vi "synchronization_prototype.vi"() -> ()   [LabVIEW 2015]
uses:
  <vilib>/userdefined/High Color/nirio_resource_hc.ctl
  FPGA_Controls/trigger_channel.ctl
  <vilib>/DAQmx/read.llb/DAQmx Read (Analog Wfm 1Chan NSamp).vi
  <vilib>/Utility/error.llb/Error Cluster From Error Code.vi
  <vilib>/rvi/errors/niLvFpgaAdjustHostInterfaceError.vi
  <vilib>/DAQmx/create/channels.llb/DAQmx Create Channel (AI-Voltage-Basic).vi
  <vilib>/DAQmx/configure/timing.llb/DAQmx Timing (Sample Clock).vi
  <vilib>/DAQmx/create/channels.llb/DAQmx Create Channel (CO-Pulse Generation-Time).vi
  <vilib>/DAQmx/configure/timing.llb/DAQmx Timing (Implicit).vi
  <vilib>/DAQmx/configure/trigger.llb/DAQmx Start Trigger (Digital Edge).vi
  <instrlib>/niSync/niSync.llb/niSync Initialize (IVI).vi
  <vilib>/DAQmx/miscellaneous.llb/DAQmx Fill In Error Info.vi
  <vilib>/FPGAPlugInAG/Dynamic/niLvFpga_Close_Dynamic.vi
  <vilib>/rvi/interface/nirviReadWriteControl/nirviReadWriteControl.xnode
  <vilib>/rvi/interface/nirviCloseFPGA/nirviCloseFPGA.xnode
  <resource>/objmgr/daqmx.rc
  <vilib>/rvi/interface/Simulation/niFpgaSimulationCallBeginRW.vi
  NiFpgaLv.dll
panel:
  in  "Pulse delay":dbl=1e-05 format="%#_13g"
  in  "Pulse counter destination terminal":string(combo)="PXI_Trig1"
  in  "DAQ pulse gen looking at:":tag
  in  "DAQ pulse gen counter":tag
  in  "DAQ Physical Channel":tag
  in  "samples DAQ":i32=1000
  in  "FPGA AI to plot":i32
  out "RIO":waveform(dbl)(graph)
  out "Interleaved Raw Data":u64[](array[numeric])
  out "Counts":i16[][](array[numeric])
  out "Voltage":dbl[][](array[numeric])
  in  "Trigger Channel FPGA looks at":T1
  in  "FPGA delay (x 50ns)":u64
  in  "num samples RIO":u64=1000
  in  "FPGA name":T2 caption="RIO Device"
  out "DAQ":waveform(dbl)(graph)
  in  "DAQ listens to":tag
  in  "DAQ Delay (s)":dbl
  in  "RIO Destination Terminal":string(combo)="PXI_Trig1"
  in  "DAQ destination terminal":string(combo)="PXI_Trig1"
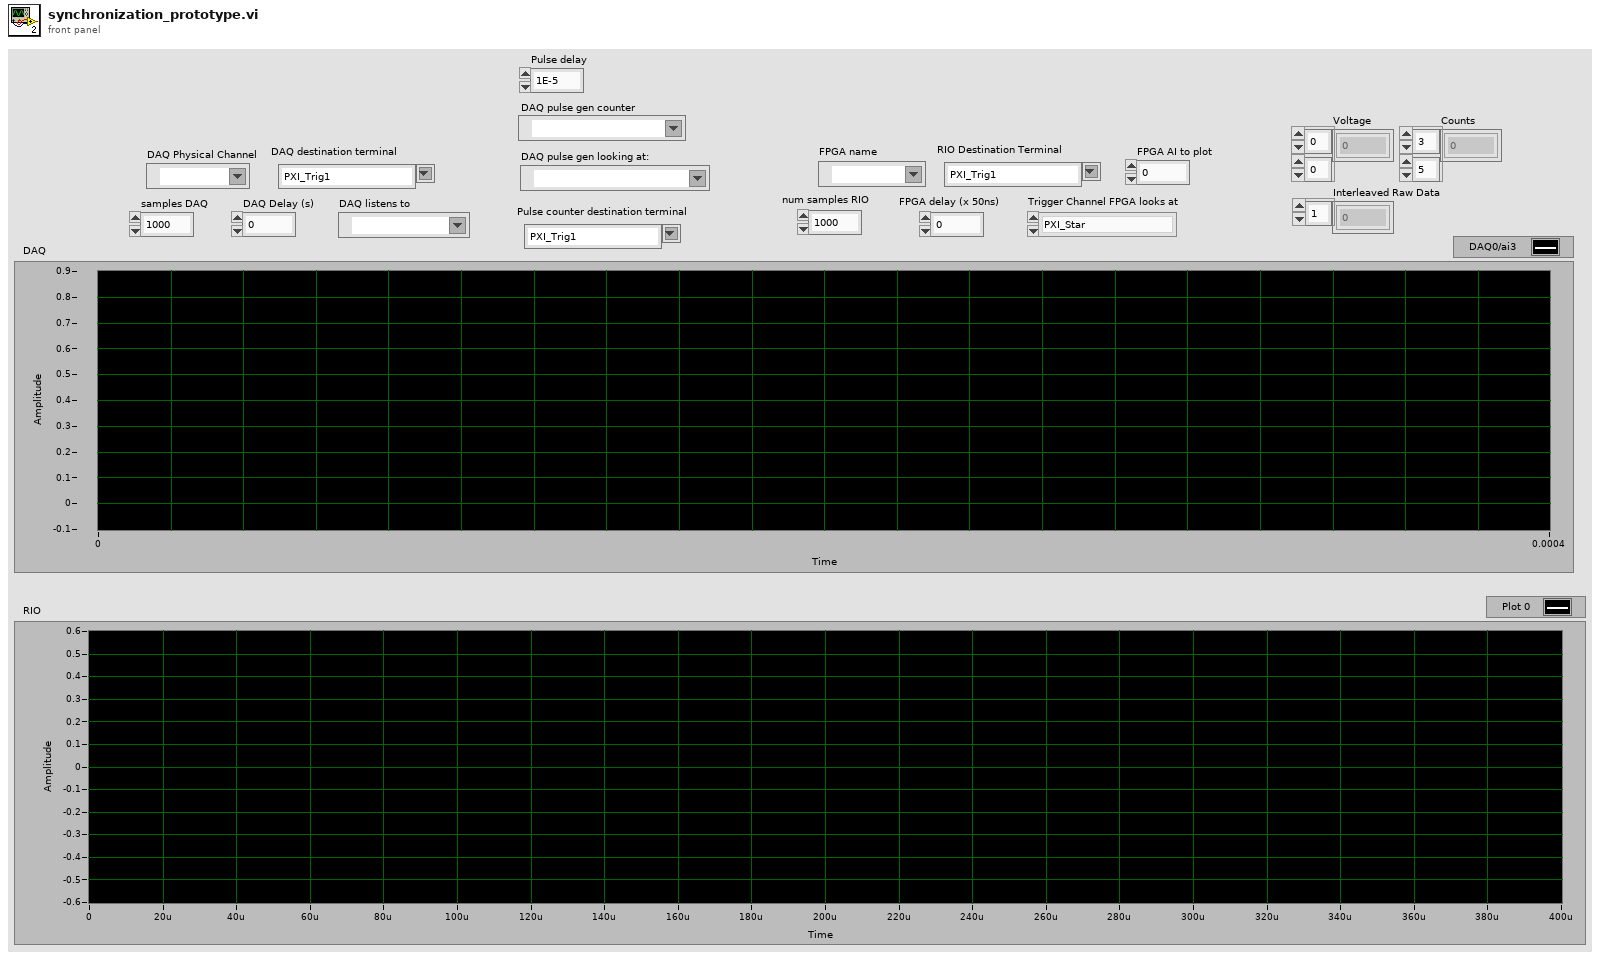
[diagram p1: front panel]
types:
  T1 = typedef "trigger_channel.ctl" = enum16{"PXI_Star", "PXI_Trig0", "PXI_Trig1", "PXI_Trig2", "PXIe_DStarB", "False", "True"}
  T2 = typedef "nirio_resource_hc.ctl" = tag
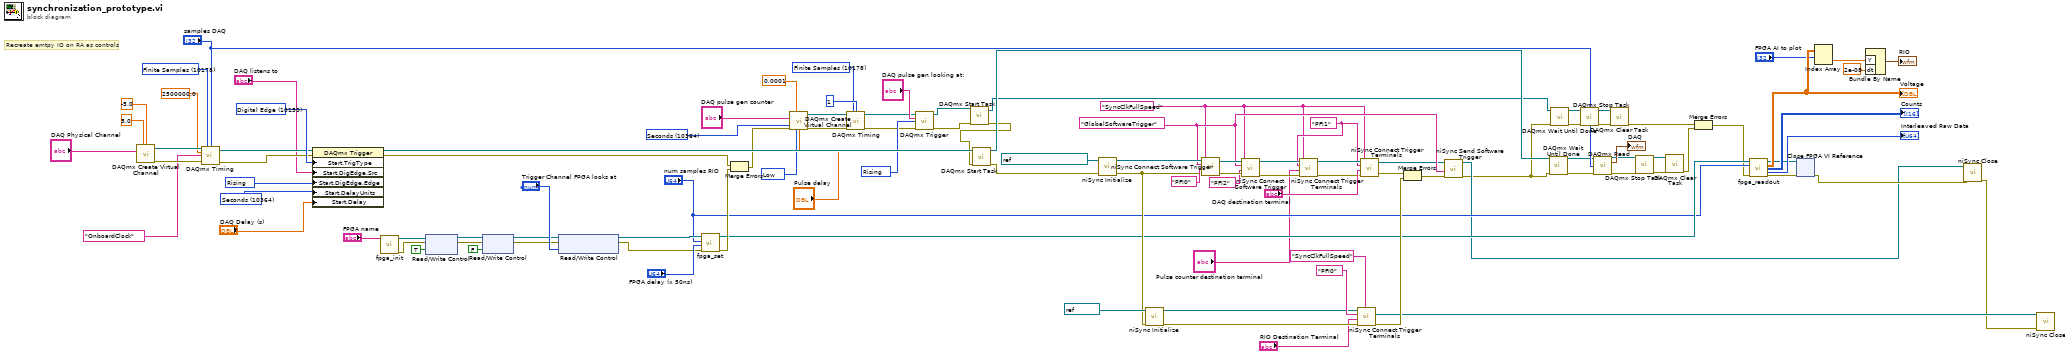
[diagram p0: block diagram]
diagram:
  w20 = 10178 items=["Finite Samples"=10178, "Continuous Samples"=10123, "Hardware Timed Single Point"=12522] ("sample mode")
  w26 = 10280 items=["Rising"=10280, "Falling"=10171] ("edge")
  w28 = 10364 items=["Seconds"=10364] ("units")
  w29 = 10214 items=["High"=10192, "Low"=10214] ("idle state")
  w73 = 10280 items=["Rising"=10280, "Falling"=10171] ("Start.DigEdge.Edge")
  w78 = 10364 items=["Sample Clock Periods"=10286, "Seconds"=10364, "Ticks"=10304] ("Start.DelayUnits")
  w79 = 10150 items=["Analog Edge"=10099, "Digital Edge"=10150, "Digital Pattern"=10398, "Analog Window"=10103, "None"=10230] ("Start.TrigType")
  w81 = 10178 items=["Finite Samples"=10178, "Continuous Samples"=10123, "Hardware Timed Single Point"=12522] ("sample mode")
  w3 = "PFI1" ("source terminal")
  w2 = "SyncClkFullSpeed" ("synchronization clock")
  w92 = "GlobalSoftwareTrigger" ("source terminal")
  # "Recreate emtpy IO on RA as controls"
  n1 = call-poly <vilib>:"DAQmx Create Virtual Channel.vi"("maximum value"=5.0, "minimum value"=-5.0, "physical channels"="DAQ Physical Channel") -> ("task out"=w85:refnum<k21>, "error out"=w84:errorcluster)  [unwired: 11 in]
  n2 = call-poly <vilib>:"DAQmx Timing.vi"("task/channels in"=w85, "sample mode"=w81, "samples per channel"="samples DAQ", "rate"=2500000.0, "source"=tag "OnboardClock", "error in"=w84) -> ("task out"=w76:refnum<k21>, "error out"=w75:errorcluster)  [unwired: 8 in]
  n3 = property class="DAQmx Trigger"(reference=w76, error in=w75, "Start.TrigType"=w79, "Start.DigEdge.Src"="DAQ listens to", "Start.DigEdge.Edge"=w73, "Start.DelayUnits"=w78, "Start.Delay"="DAQ Delay (s)") -> (reference out=w71:refnum<k21>, error out=w47:errorcluster)
  n4 = call "fpga_init.vi"("FPGA name"="FPGA name") -> ("error out"=w58:errorcluster, "FPGA VI Reference Out"=w59:refnum<k20>)  [unwired: 9 in]
  n5 = xnode "Read/Write Control"("FPGA VI Reference In"=w59, "error in"=w58, "clear"=TRUE) -> ("FPGA VI Reference Out"=w40:refnum<k20>, "error out"=w39:errorcluster)
  n6 = xnode "Read/Write Control"("FPGA VI Reference In"=w40, "error in"=w39, "clear"=FALSE) -> ("FPGA VI Reference Out"=w37:refnum<k20>, "error out"=w38:errorcluster)
  n7 = xnode "Read/Write Control"("FPGA VI Reference In"=w37, "error in"=w38, "Trigger Channel"="Trigger Channel FPGA looks at") -> ("FPGA VI Reference Out"=w62:refnum<k20>, "error out"=w61:errorcluster)
  n8 = call "fpga_set.vi"("error in"=w61, "trigger  delay"="FPGA delay (x 50ns)", "num samples"="num samples RIO", "FPGA VI Reference In"=w62) -> ("error out"=w46:errorcluster, "FPGA VI Reference Out"=w44:refnum<k20>)  [unwired: 6 in]
  n9 = Merge Errors(w47, w46) -> (w32:errorcluster)
  n10 = call-poly <vilib>:"DAQmx Create Virtual Channel.vi"("high time"=0.0001, "counter"="DAQ pulse gen counter", "units"=w28, "error in"=w32, "idle state"=w29, "initial delay"="Pulse delay") -> ("task out"=w25:refnum<k21>, "error out"=w23:errorcluster)  [unwired: 8 in]
  n11 = call-poly <vilib>:"DAQmx Timing.vi"("task/channels in"=w25, "sample mode"=w20, "samples per channel"=1, "error in"=w23) -> ("task out"=w24:refnum<k21>, "error out"=w22:errorcluster)  [unwired: 10 in]
  n12 = call-poly <vilib>:"DAQmx Trigger.vi"("task/channels in"=w24, "source"="DAQ pulse gen looking at:", "edge"=w26, "error in"=w22) -> ("task out"=w17:refnum<k21>, "error out"=w19:errorcluster)  [unwired: 10 in]
  n13 = call <vilib>:"DAQmx Start Task.vi"("task/channels in"=w17, "error in"=w19) -> ("task out"=w12:refnum<k21>, "error out"=w18:errorcluster)  [unwired: 12 in]
  n14 = call <vilib>:"DAQmx Start Task.vi"("task/channels in"=w71, "error in"=w18) -> ("task out"=w35:refnum<k21>, "error out"=w72:errorcluster)  [unwired: 12 in]
  n15 = call-poly <instrlib>:"niSync Initialize.vi"("error in (no error)"=w72, "resource name"=refnum<k15> "Sync") -> ("error out"=w80:errorcluster, "instrument handle out"=w106:refnum<k15>)  [unwired: 1 in, 7 out]
  n16 = call-poly <instrlib>:"niSync Initialize.vi"("error in (no error)"=w80, "resource name"=refnum<k15> "Sync1") -> ("error out"=w101:errorcluster, "instrument handle out"=w97:refnum<k15>)  [unwired: 1 in, 7 out]
  n17 = call <instrlib>:"niSync Connect Software Trigger.vi"("synchronization clock"=w2, "error in (no error)"=w80, "destination terminal"="PFI0", "source terminal"=w92, "instrument handle"=w106) -> ("error out"=w103:errorcluster, "instrument handle out"=w104:refnum<k15>)  [unwired: 2 in, 3 out]
  n18 = call <instrlib>:"niSync Connect Software Trigger.vi"("synchronization clock"=w2, "error in (no error)"=w103, "destination terminal"="PFI2", "source terminal"=w92, "instrument handle"=w104) -> ("error out"=w5:errorcluster, "instrument handle out"=w7:refnum<k15>)  [unwired: 2 in, 3 out]
  n19 = call <instrlib>:"niSync Connect Trigger Terminals.vi"("synchronization clock"=w2, "error in (no error)"=w5, "destination terminal"="Pulse counter destination terminal", "source terminal"=w3, "instrument handle"=w7) -> ("error out"=w4:errorcluster, "instrument handle out"=w6:refnum<k15>)  [unwired: 5 in]
  n20 = call <instrlib>:"niSync Connect Trigger Terminals.vi"("synchronization clock"="SyncClkFullSpeed", "error in (no error)"=w101, "destination terminal"="RIO Destination Terminal", "source terminal"="PFI0", "instrument handle"=w97) -> ("error out"=w98:errorcluster, "instrument handle out"=w90:refnum<k15>)  [unwired: 5 in]
  n21 = call <instrlib>:"niSync Connect Trigger Terminals.vi"("synchronization clock"=w2, "error in (no error)"=w4, "destination terminal"="DAQ destination terminal", "source terminal"=w3, "instrument handle"=w6) -> ("error out"=w96:errorcluster, "instrument handle out"=w91:refnum<k15>)  [unwired: 5 in]
  n22 = Merge Errors(w96, w98) -> (w93:errorcluster)
  n23 = call <instrlib>:"niSync Send Software Trigger.vi"("error in (no error)"=w93, "source terminal"=w92, "instrument handle"=w91) -> ("error out"=w11:errorcluster, "instrument handle out"=w42:refnum<k15>)  [unwired: 7 out]
  n24 = call <vilib>:"DAQmx Wait Until Done.vi"("task/channels in"=w35, "error in"=w11) -> ("task out"=w36:refnum<k21>, "error out"=w34:errorcluster)  [unwired: 12 in]
  n25 = call <vilib>:"DAQmx Wait Until Done.vi"("task/channels in"=w12, "error in"=w11) -> ("task out"=w14:refnum<k21>, "error out"=w13:errorcluster)  [unwired: 12 in]
  n26 = call <vilib>:"DAQmx Stop Task.vi"("task/channels in"=w14, "error in"=w13) -> ("task out"=w15:refnum<k21>, "error out"=w16:errorcluster)  [unwired: 12 in]
  n27 = call-poly <vilib>:"DAQmx Read.vi"("task/channels in"=w36, "number of samples per channel"="samples DAQ", "error in"=w34) -> ("task out"=w68:refnum<k21>, "data"=→"DAQ":waveform(dbl), "error out"=w69:errorcluster)  [unwired: 10 in]
  n28 = call <vilib>:"DAQmx Clear Task.vi"("task in"=w15, "error in"=w16) -> ("error out"=w10:errorcluster)  [unwired: 13 in]
  n29 = call <vilib>:"DAQmx Stop Task.vi"("task/channels in"=w68, "error in"=w69) -> ("task out"=w66:refnum<k21>, "error out"=w65:errorcluster)  [unwired: 12 in]
  n30 = call <vilib>:"DAQmx Clear Task.vi"("task in"=w66, "error in"=w65) -> ("error out"=w9:errorcluster)  [unwired: 13 in]
  n31 = Merge Errors(w10, w9) -> (w8:errorcluster)
  n32 = call "fpga_readout.vi"("FPGA VI Reference In"=w44, "samples"="num samples RIO", "error in"=w8) -> ("FPGA Reference Out"=w45:refnum<k20>, "Voltage"=w50:dbl[][], "Counts"=→"Counts":i16[][], "Interleaved Raw Data"=→"Interleaved Raw Data":u64[], "error out"=w56:errorcluster)  [unwired: 8 in]
  "Voltage" <- w50
  n33 = xnode "Close FPGA VI Reference"("FPGA VI Reference In"=w45, "error in"=w56) -> ("error out"=w48:errorcluster)
  n34 = Index Array(array=w50, index (row)="FPGA AI to plot") -> (element=w54:dbl[])  [unwired: 1 in]
  n35 = Bundle By Name("Y"=w54, "dt"=2e-08) -> (→"RIO":waveform(dbl))  [unwired: 1 in]
  n36 = call <instrlib>:"niSync Close.vi"("error in (no error)"=w48, "instrument handle"=w42) -> ("error out"=w89:errorcluster)  [unwired: 9 out]
  n37 = call <instrlib>:"niSync Close.vi"("error in (no error)"=w89, "instrument handle"=w90) -> ()  [unwired: 10 out]
